vi "TEST_PP_CmdSend_End.vi"() -> ()   [LabVIEW 2023]
uses:
  <vilib>/Rock Robotics/WPI/ThirdParty/JAS_Junk/TrajLib/VI/BoolCmd_Recv_Internal.vi
  <vilib>/Rock Robotics/WPI/ThirdParty/JAS_Junk/TrajLib/VI/BoolCmd_Send_Internal.vi
  <vilib>/Rock Robotics/WPI/ThirdParty/JAS_Junk/TrajLib/VI/DigSeqLogic_Edge_On.vi
  <vilib>/Rock Robotics/WPI/ThirdParty/JAS_Junk/TrajLib/VI/BoolCmd_ObtainQueue.vi
  <vilib>/Rock Robotics/WPI/ThirdParty/JAS_Junk/TrajLib/Trajectory_Library.lvlib
panel:
  in  "s":bool
  in  "Ready1":bool=TRUE
  out "Do Command 1":bool
  out "Do Command 2":bool
  out "Do Cancel":bool
  in  "Ready2":bool=TRUE
  in  "Boolean 2":bool
  in  "Boolean":bool
  out "Receive End":bool
  out "New Request":bool
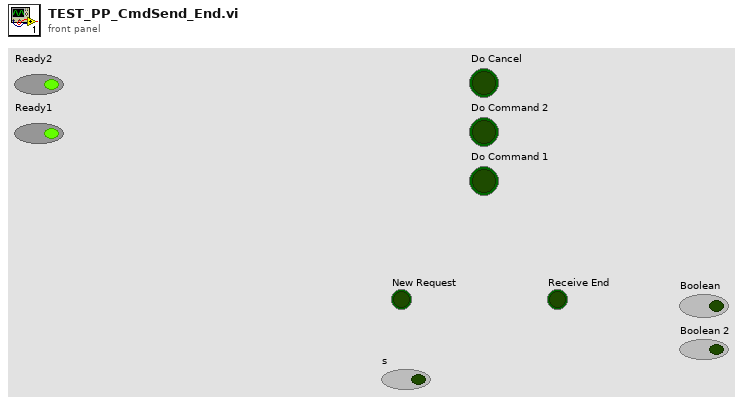
[diagram p1: front panel]
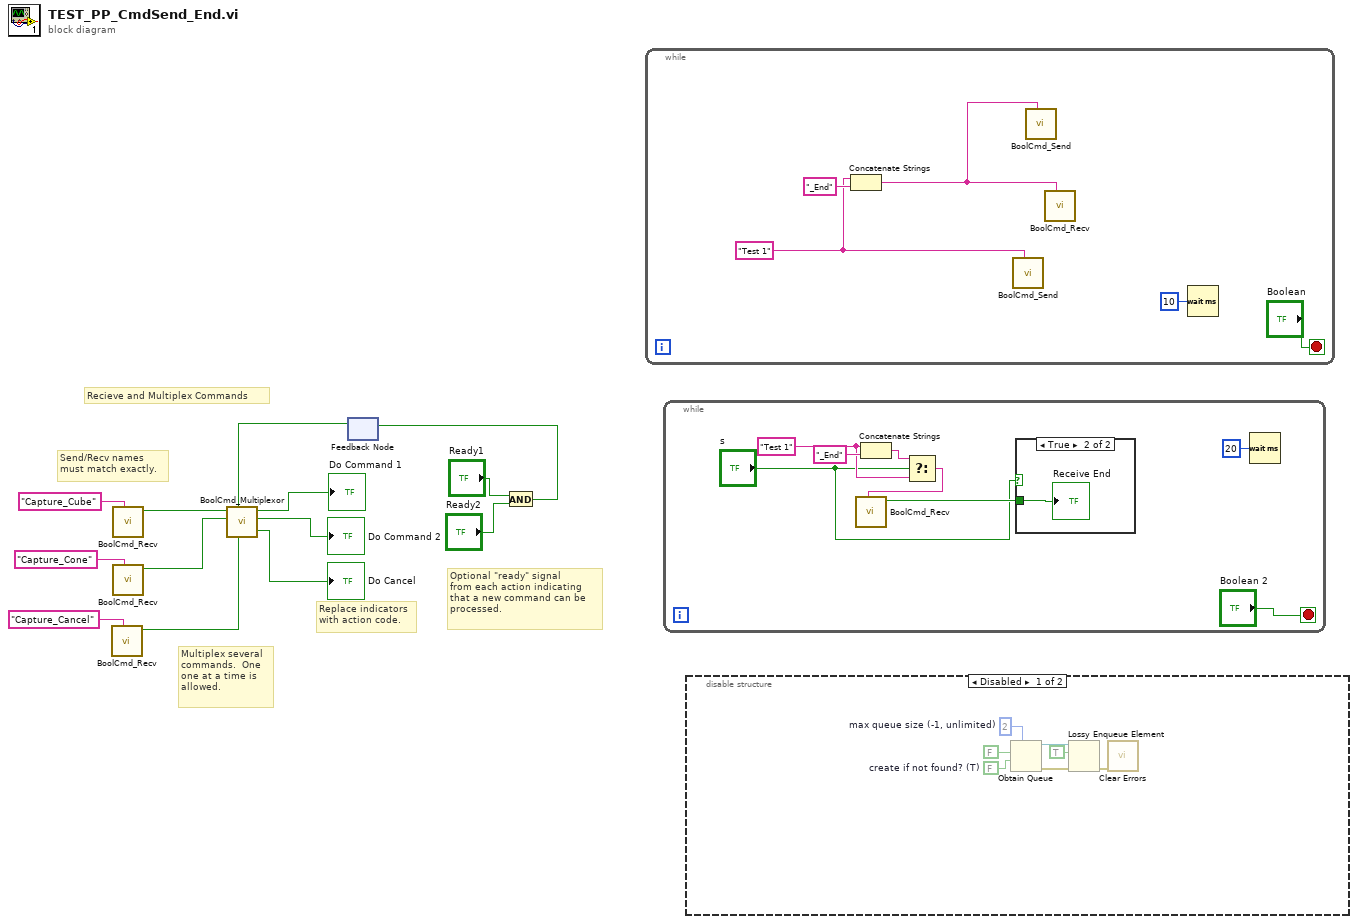
[diagram p0: block diagram]
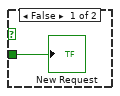
[diagram p3: hidden frame]
diagram:
  # "Replace indicators\nwith action code."
  # "Optional \"ready\" signal\nfrom each action indicating\nthat a new command can be\nprocessed."
  # "Multiplex several\ncommands.  One\none at a time is \nallowed."
  # "Send/Recv names\nmust match exactly."
  # "Recieve and Multiplex Commands"
  n1 = call <vilib>:"BoolCmd_Recv.vi"("Command Name"="Capture_Cancel") -> ("New Request"=w6:bool)  [unwired: 9 in, 1 out]
  n2 = call <vilib>:"BoolCmd_Recv.vi"("Command Name"="Capture_Cube") -> ("New Request"=w4:bool)  [unwired: 9 in, 1 out]
  n3 = call <vilib>:"BoolCmd_Recv.vi"("Command Name"="Capture_Cone") -> ("New Request"=w5:bool)  [unwired: 9 in, 1 out]
  n4 = feedback #1() -> (w13:bool)  [unwired: 1 in]
  n5 = call <vilib>:"BoolCmd_Multiplexor.vi"("Command Cancel"=w6, "Ready"=w13, "Command 2"=w5, "Command 1"=w4) -> ("Do Command 2"=→"Do Command 2":bool, "Do Command 1"=→"Do Command 1":bool, "Do Cancel"=→"Do Cancel":bool)  [unwired: 3 in, 2 out]
  n6 = And(x="Ready1", y="Ready2") -> (x .and. y?=w12:bool)
  n7 = feedback-in #1(w12) -> ()
  n8 = while {
    stop <- "Boolean" stop-if-true
    w16 = "Test 1" ("name (unnamed)")
    n9 = Concatenate Strings(w16, "_End" ("string")) -> (w14:string)
    n10 = call <vilib>:"BoolCmd_Send.vi"("Command Name"=w16) -> ()  [unwired: 10 in, 1 out]
    n11 = call <vilib>:"BoolCmd_Send.vi"("Command Name"=w14) -> ()  [unwired: 10 in, 1 out]
    n12 = call <vilib>:"BoolCmd_Recv.vi"("Command Name"=w14) -> ()  [unwired: 9 in, 2 out]
    n13 = Wait (ms)(milliseconds to wait=u32 10) -> ()  [unwired: 1 out]
  }
  n14 = while {
    stop <- "Boolean 2" stop-if-true
    w22 = "Test 1" ("name (unnamed)")
    n15 = Concatenate Strings(w22, "_End" ("string")) -> (w23:string)
    n16 = Select(t=w23, s="s", f=w22) -> (s? t:f=w21:string)
    n17 = call <vilib>:"BoolCmd_Recv.vi"("Command Name"=w21) -> ("New Request"=w20:bool)  [unwired: 9 in, 1 out]
    n18 = case shown="True" "s" {
      tunnel: w20 -> [w27 w28]
      frame False {
        "New Request" <- w27
      }
      frame True {
        "Receive End" <- w28
      }
    }
    n19 = Wait (ms)(milliseconds to wait=u32 20) -> ()  [unwired: 1 out]
  }
  n20 = disable-structure shown="Disabled" {
    frame Disabled {
      w35 = FALSE  # create if not found? (T)
      w36 = 2  # max queue size (-1, unlimited)
      n21 = Obtain Queue(max queue size (-1, unlimited)=w36, element data type=FALSE, create if not found? (T)=w35) -> (name (unnamed)=w29:string, queue out=w32:refnum<queue>, error out=w31:errorcluster)  [unwired: 1 in, 1 out]
      n22 = Lossy Enqueue Element(queue=w32, element=TRUE, error in (no error)=w31) -> (error out=w30:errorcluster)  [unwired: 3 out]
      n23 = call <vilib>:"Clear Errors.vi"("error in (no error)"=w30) -> ()  [unwired: 5 in, 2 out]
    }
    frame Enabled {
    }
  }
